vi "CloseScanPanel.vi"(8 "error in (no error)":errorcluster caption="entrée d'erreur (pas d'erreur)", 9 "Index":i32, 10 "SubPanRef":refnum<vi>, 11 "LoadedInst":refnum<class "BaseDevice.lvclass">[](array[class])) -> (0 "sortie d'erreur":errorcluster, 3 "LoadedInst Out":refnum<class "BaseDevice.lvclass">[](array[class]) caption="LoadedInst")   [LabVIEW 2019, in "BaseDevice.lvclass"]
uses:
  BaseDevice.lvclass
  BaseDevice.lvclass/BaseDevice.ctl
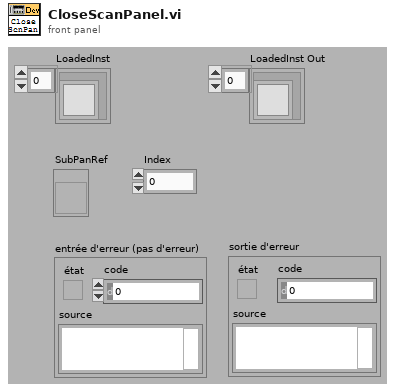
[diagram p1: front panel]
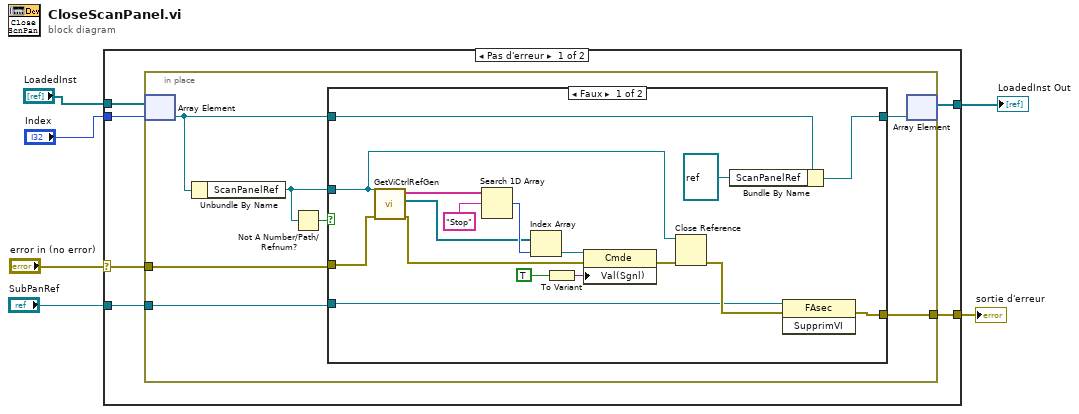
[diagram p0: block diagram]
diagram:
  n1 = case shown="Pas d'erreur" "error in (no error)" {
    selector: "error in (no error)" -> [w12 w40]
    tunnel: [w11 w40] -> w5
    tunnel: "SubPanRef" -> [w10 _]
    tunnel: [w9 w39] -> w3
    tunnel: "LoadedInst" -> [w8 w39]
    tunnel: "Index" -> [w7 _]
    frame No Error {
      n2 = in-place {
        in-place-border: w12 -> [w19]
        in-place-border: [w18] -> w11
        in-place-border: w10 -> [w15]
        n3 = in-place-array #1(w8, w7) -> (w17:refnum<class "BaseDevice.lvclass">)
        n4 = Unbundle By Name(w17) -> ("ScanPanelRef"=w13:refnum<vi>)
        n5 = Not A Number/Path/Refnum?(number/path/refnum=w13) -> (NaN/Path/Refnum?=w14:bool)
        n6 = case shown="Faux" w14 {
          tunnel: w19 -> [w36 w37]
          tunnel: [w35 w37] -> w18
          tunnel: w13 -> [w23 _]
          tunnel: w17 -> [w22 w38]
          tunnel: [w21 w38] -> w16
          tunnel: w15 -> [w20 _]
          frame False {
            n7 = call <userlib>:"GetViCtrlRefGen.vi"("ErrorIn(No Error)"=w36, "VIRef"=w23) -> ("sortie d'erreur"=w29:errorcluster, "ControlsRefs"=w32:refnum<vi>[], "ControlsNames"=w34:string[])  [unwired: 7 in]
            n8 = Search 1D Array(1D array=w34, element="Stop") -> (index of element=w33:i32)  [unwired: 1 in]
            n9 = Index Array(array=w32, index=w33) -> (element=w30:refnum<vi>)
            n10 = To Variant(anything=TRUE) -> (Variant=w27:variant)
            n11 = property class="Cmde"(reference=w30, error in=w29, "Val(Sgnl)"=w27) -> (error out=w26:errorcluster)  [unwired: 1 out]
            n12 = Close Reference(reference=w23, error in (no error)=w26) -> (error out=w24:errorcluster)
            n13 = Bundle By Name(cluster=w22, "ScanPanelRef"=refnum<vi> refnum) -> (w21:refnum<class "BaseDevice.lvclass">)
            n14 = invoke class="FAsec" method="SupprimVI"(reference=w20, error in=w24) -> (error out=w35:errorcluster)  [unwired: 1 in, 2 out]
          }
          frame True {
          }
        }
        n15 = in-place-array #1(w16) -> (w9:refnum<class "BaseDevice.lvclass">[])  [unwired: 1 out]
      }
    }
    frame Error {
    }
  }
  "sortie d'erreur" <- w5
  "LoadedInst Out" <- w3
